vi "DWF PS Initialize.vi"(0 "Device Name":string, 5 "Reset":bool=TRUE caption="Reset (True)", 11 "Error In":errorcluster caption="Error In (no error)") -> (4 "Instrument Handle Out":u32, 15 "Error Out":errorcluster)   [LabVIEW 2015, in "DigilentWF.lvlib"]
doc: "Establishes communication with the device. This VI should be called once per session."
uses:
  <vilib>/DigilentWF/DigilentWF.lvlib
  dwf.dll
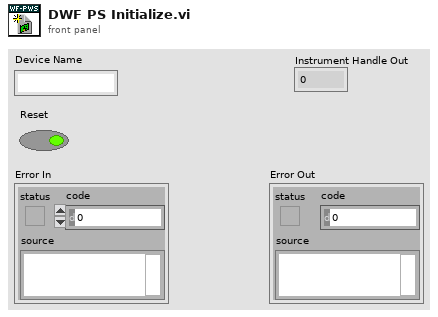
[diagram p1: front panel]
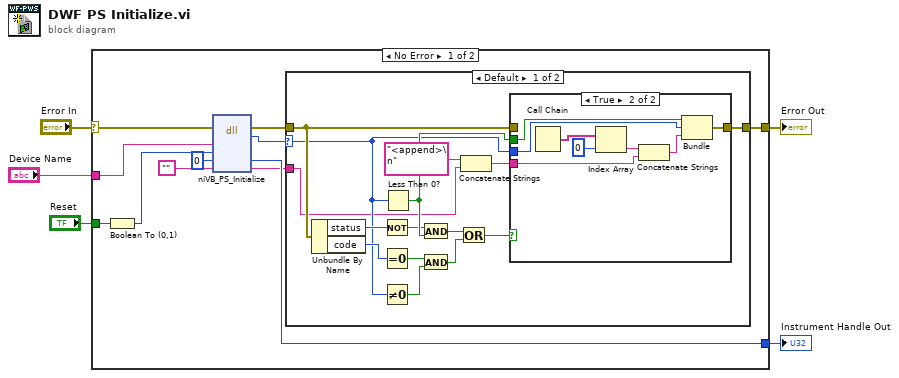
[diagram p0: block diagram]
diagram:
  n1 = case "outter_case" shown="No Error" "Error In" {
    selector: "Error In" -> [w14 w42]
    tunnel: [w16 w42] -> w4
    tunnel: "Device Name" -> [w12 _]
    tunnel: "Reset" -> [w15 _]
    tunnel: [w9 _] -> w1
    frame No Error {
      n2 = Boolean To (0,1)(Boolean=w15) -> (0, 1=w11:i16)
      n3 = dll-call lib="dwf.*" fn="niVB_PS_Initialize"(error in=w14, "deviceName"=w12, "reset"=w11, "instrumentHandle"=u64 0, "szError"="") -> (error out=w13:errorcluster, "return type"=w10:i32, "instrumentHandle"=w9:u64, "szError"=w7:string)  [unwired: 4 in, 1 out]
      n4 = case "inner_case" shown="Default" w10 {
        selector: w10 -> [w21 _]
        tunnel: w13 -> [w22 w41]
        tunnel: [w18 w41] -> w16
        tunnel: w7 -> [w17 _]
        frame Default {
          n5 = Unbundle By Name(w22) -> ("status"=w26:bool, "code"=w30:i32)
          n6 = Not(x=w26) -> (.not. x?=w29:bool)
          n7 = Equal To 0?(x=w30) -> (x = 0?=w25:bool)
          n8 = Not Equal To 0?(x=w21) -> (x != 0?=w28:bool)
          n9 = Less Than 0?(x=w21) -> (x < 0?=w31:bool)
          n10 = And(x=w29, y=w31) -> (x .and. y?=w27:bool)
          n11 = And(x=w25, y=w28) -> (x .and. y?=w24:bool)
          n12 = Or(x=w27, y=w24) -> (x .or. y?=w23:bool)
          n13 = Concatenate Strings("<append>\n" ("string"), w17) -> (w20:string)
          n14 = case shown="True" w23 {
            tunnel: [w32 w39] -> w18
            tunnel: w21 -> [_ w38]
            tunnel: w31 -> [_ w37]
            tunnel: w22 -> [w32 _]
            tunnel: w20 -> [_ w33]
            frame False {
            }
            frame True {
              n15 = Call Chain() -> (call chain=w36:string[])
              n16 = Index Array(array=w36, index=0) -> (element=w35:string)
              n17 = Concatenate Strings(w35, w33) -> (w40:string)
              n18 = Bundle(w37, "return type"=w38, w40) -> (w39:cluster{bool, "return type":i32, string})  [unwired: 1 out]
            }
          }
        }
        frame 0 {
        }
      }
    }
    frame Error {
    }
  }
  "Error Out" <- w4
  "Instrument Handle Out" <- w1
